vi "BrightfieldControl.vi"() -> ()   [LabVIEW 2019]
doc: "high-level user control for uc480/ThorCam DCx camera. include MouseMove, this allows mouse click to move stage motor capabilities"
uses:
  <vilib>/Utility/miscctls.llb/LVPoint32TypeDef.ctl
  C:/Program Files/Thorlabs/Scientific Imaging/DCx Camera Support/Develop/DotNet/uc480DotNet.dll
  System.Drawing
  System.Windows.Forms
panel:
  out "Coords":T1
  out "# in queue":i32
  in  "motor move?":bool
  out "mouse click":string
  out "mm value w":dbl
  out "mm value h":dbl
  in  "micron/pixel":dbl=2.0
  in  "stop video loop":bool
  out "current video state":string="wait for init"
  in  "save video?":bool
  in  "mode":i32(ring)=128 items=["BGRA8Packed"=0, "BGR8Packed"=1, "BGR565Packed"=2, "BGR5Packed"=3, "Mono8"=6, "SensorRaw8"=11, "UYVYPacked"=12, "UYVYMonoPacked"=13, "UYVYBayerPacked"=14, "CBYCRYPacked"=23, "BGRY8Packed"=24, "BGR10Packed"=25, "Mono12"=26, "SensorRaw12"=27, "Mono16"=28, "SensorRaw16"=29, "BGR12Unpacked"=30, "BGRA12Unpacked"=31, "Jpeg"=32, "SensorRaw10"=33, "Mono10"=34, "BGR10Unpacked"=35, "RGBA8Packed"=128, "RGB8Packed"=129, "RGBY8Packed"=152, "RGB10Packed"=153, "RGB12Unpacked"=158, "RGBA12Unpacked"=159, "RGB10Unpacked"=163, "RGB8Planar"=8321, "PreferPackedSourceFormat"=16384]
  out "img saved to:":string
  in  "Folder path save":path
  in  "PictureBox":refnum<k24>(container)
  in  "Stop Button":bool
  in  "Image filename save":string="D:\\Victor Sun\\optical trap control\\output_test\\test"
  in  "save snapshot?":bool
  in  "Pixelclock":i32(slide)=24 scale=5.0..43.0
  in  "Framerate":dbl(slide)=7.0 scale=5.0..14.0
  in  "Exposure time":dbl(slide)=30.0 scale=1.0..70.0
  out "SerialNumber":string
  in  "s32Cam":i32
  # "MouseMove"
  # "trying to figure out to use .net video \nto get .avi"
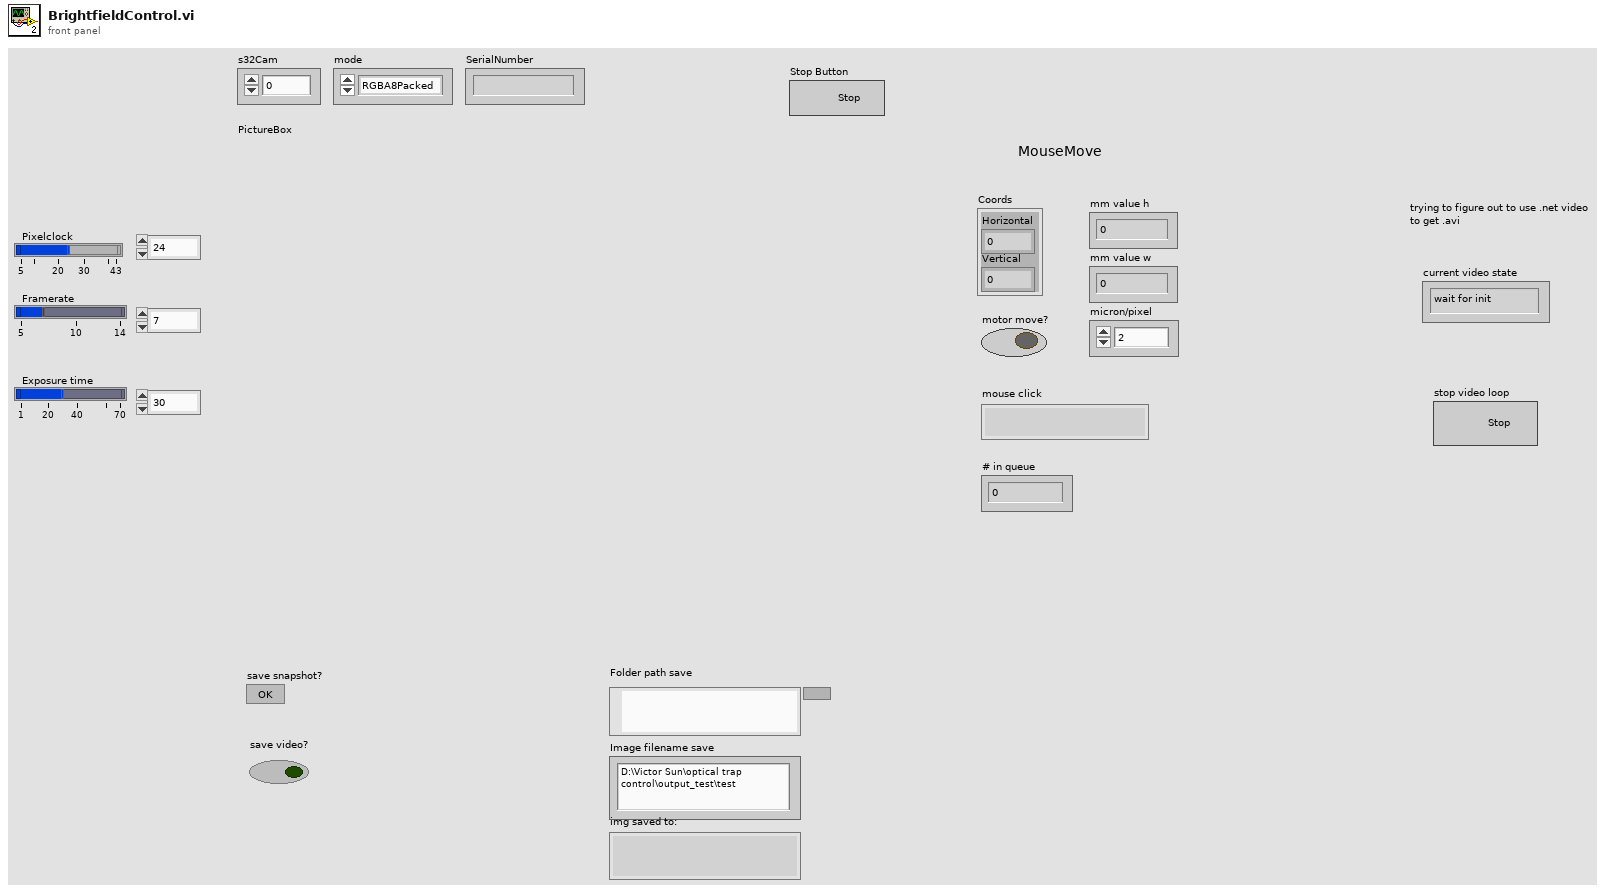
[diagram p1: front panel]
types:
  T1 = typedef "LVPoint32TypeDef.ctl" = cluster{"Horizontal":i32, "Vertical":i32}
  T2 = enum16{"wait for init", "init video", "wait for write", "write frame", "close video"}
  T3 = typedef "IMAQ AVI2 Refnum.ctl" = refnum<k20>
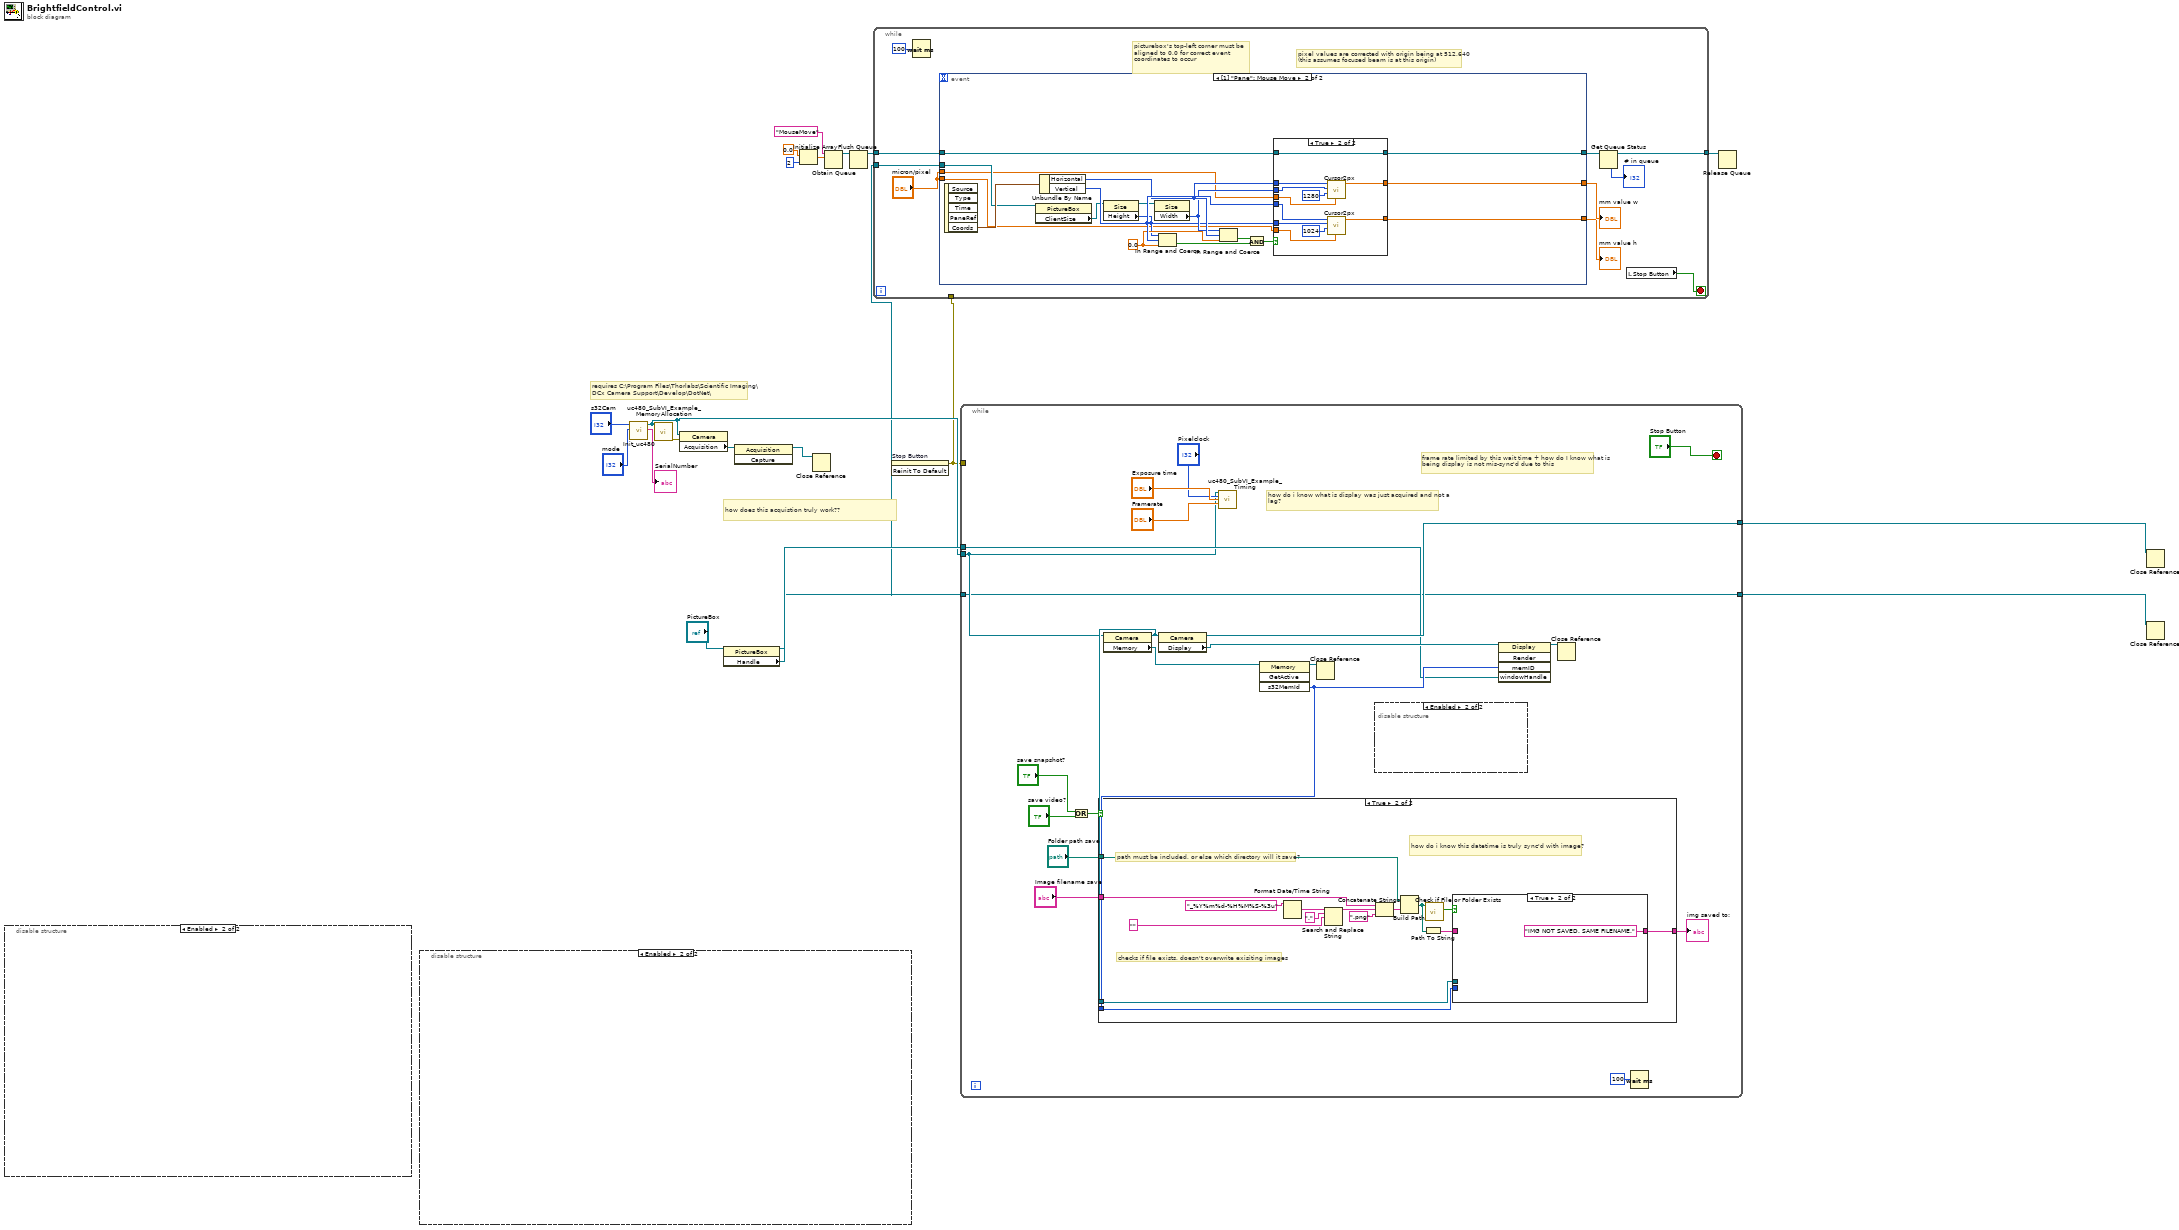
[diagram p0: block diagram]
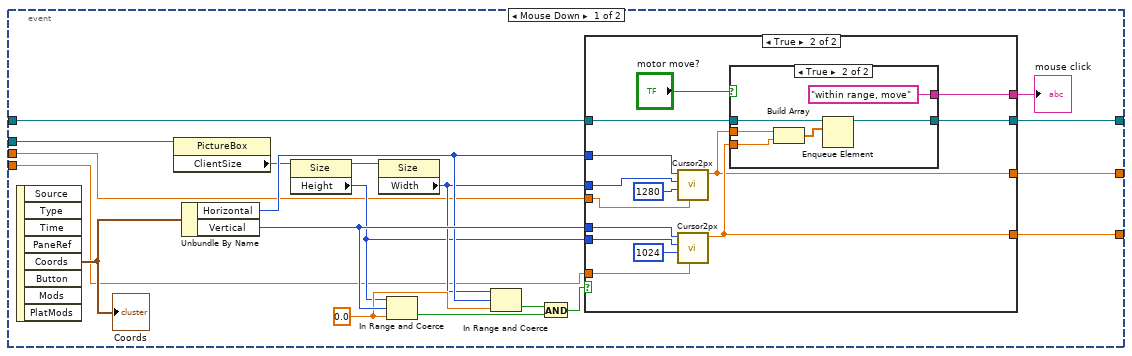
[diagram p2: hidden frame]
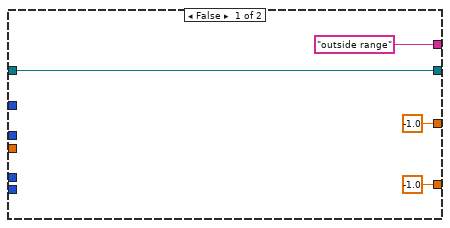
[diagram p3: hidden frame]
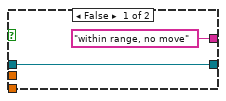
[diagram p4: hidden frame]
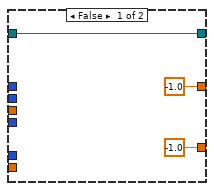
[diagram p5: hidden frame]
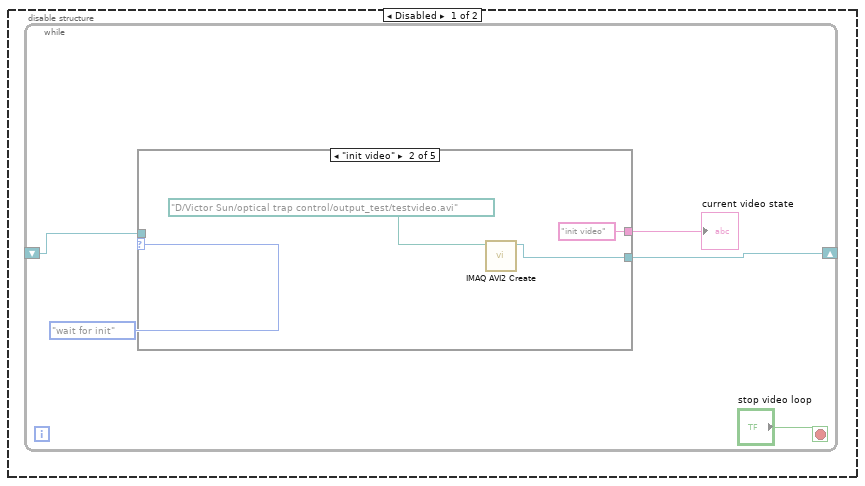
[diagram p6: hidden frame]
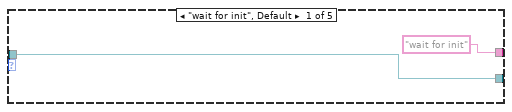
[diagram p7: hidden frame]
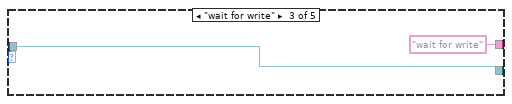
[diagram p8: hidden frame]
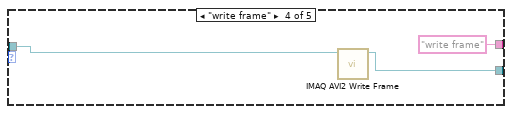
[diagram p9: hidden frame]
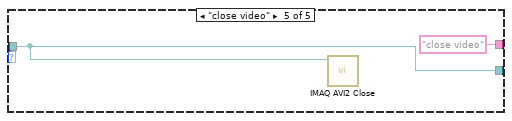
[diagram p10: hidden frame]
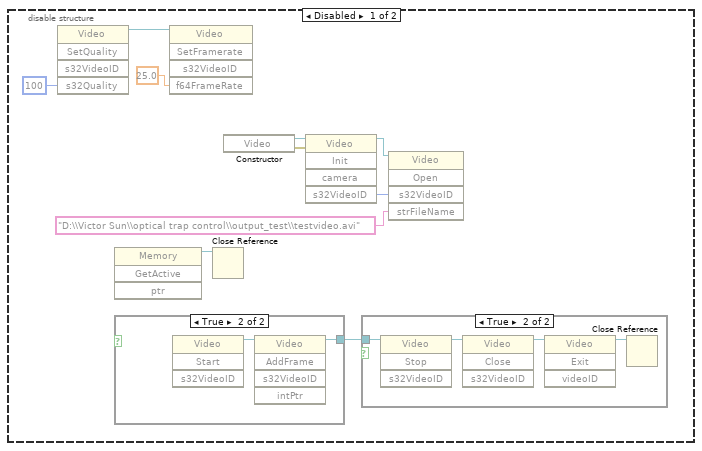
[diagram p11: hidden frame]
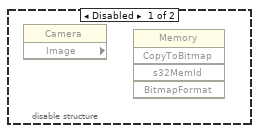
[diagram p14: hidden frame]
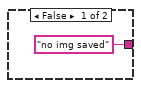
[diagram p15: hidden frame]
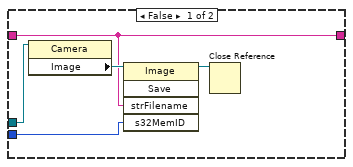
[diagram p16: hidden frame]
diagram:
  # "requires C:\\Program Files\\Thorlabs\\Scientific Imaging\\DCx Camera Support\\Develop\\DotNet\\"
  # "how does this acquistion truly work??"
  n1 = disable-structure shown="Enabled" {
    frame Disabled {
      n2 = invoke class="Video" method="SetQuality"("s32Quality"=100) -> (reference out=w25:refnum<k24>)  [unwired: 4 in, 4 out]
      n3 = invoke class="Memory" method="GetActive"() -> (reference out=w22:refnum<k24>)  [unwired: 4 in, 3 out]
      n4 = case shown="True" {
        selector: _ -> [_ _]
        tunnel: [_ w35] -> w21
        frame False {
        }
        frame True {
          n5 = invoke class="Video" method="Start"() -> (reference out=w36:refnum<k24>)  [unwired: 4 in, 3 out]
          n6 = invoke class="Video" method="AddFrame"(reference=w36) -> (reference out=w35:refnum<k24>)  [unwired: 4 in, 4 out]
        }
      }
      n7 = invoke class="Video" method="SetFramerate"(reference=w25, "f64FrameRate"=25.0) -> ()  [unwired: 3 in, 5 out]
      n8 = Close Reference(reference=w22) -> ()  [unwired: 1 in, 1 out]
      n9 = constructor class="Video"() -> (reference out=w28:refnum<k24>, error out=w29:errorcluster)  [unwired: 3 in, 1 out]
      n10 = invoke class="Video" method="Init"(reference=w28, error in=w29) -> (reference out=w26:refnum<k24>, "s32VideoID"=w30:i32)  [unwired: 3 in, 3 out]
      n11 = case shown="True" {
        selector: _ -> [_ _]
        tunnel: w21 -> [_ w34]
        frame False {
        }
        frame True {
          n12 = invoke class="Video" method="Stop"(reference=w34) -> (reference out=w33:refnum<k24>)  [unwired: 3 in, 3 out]
          n13 = invoke class="Video" method="Close"(reference=w33) -> (reference out=w32:refnum<k24>)  [unwired: 3 in, 3 out]
          n14 = invoke class="Video" method="Exit"(reference=w32) -> (reference out=w31:refnum<k24>)  [unwired: 3 in, 3 out]
          n15 = Close Reference(reference=w31) -> ()  [unwired: 1 in, 1 out]
        }
      }
      n16 = invoke class="Video" method="Open"(reference=w26, "s32VideoID"=w30, "strFileName"="D:\\Victor Sun\\optical trap control\\output_test\\testvideo.avi") -> ()  [unwired: 2 in, 5 out]
    }
    frame Enabled {
    }
  }
  n17 = disable-structure shown="Enabled" {
    frame Disabled {
      n18 = while {
        shift-right: [w38] -> _
        shift-left: _ -> [w37]
        stop <- "stop video loop" stop-if-true
        n19 = case shown="\"init video\"" T2."wait for init" {
          tunnel: ["wait for init" "init video" "wait for write" "write frame" "close video"] -> w40
          tunnel: [w42 w44 w47 w49 w52] -> w38
          tunnel: w37 -> [w42 _ w47 w50 w52]
          frame "wait for init", Default {
          }
          frame "init video" {
            n20 = call "IMAQ AVI2 Create"("AVI Path"=path "D:/Victor Sun/optical trap control/output_test/testvideo.avi") -> ("AVI Refnum"=w44:T3)  [unwired: 9 in, 1 out]
          }
          frame "wait for write" {
          }
          frame "write frame" {
            n21 = call "IMAQ AVI2 Write Frame"("AVI Refnum"=w50) -> ("AVI Refnum (duplicate)"=w49:T3)  [unwired: 8 in, 2 out]
          }
          frame "close video" {
            n22 = call "IMAQ AVI2 Close"("AVI Refnum"=w52) -> ()  [unwired: 10 in, 1 out]
          }
        }
        "current video state" <- w40
      }
    }
    frame Enabled {
    }
  }
  n23 = call "Init_uc480.vi"("mode"="mode", "s32Cam"="s32Cam") -> ("SerialNumber"=→"SerialNumber":string, ".NET Refnum out"=w11:refnum<k24>)  [unwired: 8 in]
  n24 = call <instrlib>:"uc480_SubVI_Example_MemoryAllocation.vi"(".NET (Reference)"=w11) -> ("Error Out"=w12:errorcluster)  [unwired: 14 in, 4 out]
  n25 = property class="Camera"(reference=w11, error in=w12) -> ("Acquisition"=w13:refnum<k24>)  [unwired: 2 out]
  n26 = property class="PictureBox"(reference="PictureBox") -> (reference out=w9:refnum<k24>, "Handle"=w15:refnum<k24>)  [unwired: 1 in, 1 out]
  n27 = invoke class="Acquisition" method="Capture"(reference=w13) -> (reference out=w14:refnum<k24>)  [unwired: 2 in, 2 out]
  n28 = Initialize Array(0.0 ("element"), 2 ("dimension size")) -> (w5:dbl[])
  n29 = Close Reference(reference=w14) -> ()  [unwired: 1 in, 1 out]
  n30 = Obtain Queue(name (unnamed)="MouseMove", element data type=w5) -> (queue out=w3:refnum<queue>)  [unwired: 3 in, 2 out]
  n31 = Flush Queue(queue=w3) -> (queue out=w4:refnum<queue>)  [unwired: 1 in, 2 out]
  n32 = invoke on="Stop Button" class="Bool (strict)" method="Reinit To Default"() -> (error out=w1:errorcluster)  [unwired: 3 in, 2 out]
  n33 = while {
    tunnel: w9 -> [w62]
    tunnel: w4 -> [w61]
    tunnel: [w58] -> w2
    tunnel: w1 -> [_]
    stop <- w54 stop-if-true
    # "picturebox's top-left corner must be aligned to 0,0 for correct event coordinates to occur"
    # "pixel values are corrected with origin being at 512,640\n(this assumes focused beam is at this origin)"
    n34 = Wait (ms)(milliseconds to wait=u32 100) -> ()  [unwired: 1 out]
    n35 = event shown="[1] \"Pane\": Mouse Move" {
      selector: _ -> [_ _]
      dyn-events: _ -> [_ _]
      timeout: _ -> [_ _]
      tunnel: w62 -> [w72 w117]
      tunnel: w61 -> [w69 w114]
      tunnel: [w68 w113] -> w59
      tunnel: [w67 w112] -> w57
      tunnel: [w66 w111] -> w56
      tunnel: "micron/pixel" -> [w65 w110]
      tunnel: "micron/pixel" -> [w64 w109]
      event Mouse Down {
        w76 = 0.0 ("lower limit")
        n36 = event-data() -> ("Coords"=w82:T1)  [unwired: 1 in, 7 out]
        "Coords" <- w82
        n37 = property class="PictureBox"(reference=w72) -> ("ClientSize"=w73:refnum<k24>)  [unwired: 1 in, 2 out]
        n38 = Unbundle By Name(w82) -> ("Horizontal"=w77:i32, "Vertical"=w80:i32)
        n39 = property class="Size"(reference=w73) -> (reference out=w74:refnum<k24>, "Height"=w70:i32)  [unwired: 1 in, 1 out]
        n40 = property class="Size"(reference=w74) -> ("Width"=w71:i32)  [unwired: 1 in, 2 out]
        n41 = In Range and Coerce(upper limit=w70, x=w80, lower limit=w76) -> (In Range?=w79:bool)  [unwired: 1 out]
        n42 = In Range and Coerce(upper limit=w71, x=w77, lower limit=w76) -> (In Range?=w78:bool)  [unwired: 1 out]
        n43 = And(x=w78, y=w79) -> (x .and. y?=w81:bool)
        n44 = case shown="True" w81 {
          tunnel: w80 -> [_ w100]
          tunnel: w70 -> [_ w99]
          tunnel: w71 -> [_ w96]
          tunnel: w77 -> [_ w95]
          tunnel: ["outside range" ("mouse click") w93] -> w75
          tunnel: w69 -> [w85 w92]
          tunnel: [w85 w91] -> w68
          tunnel: [-1.0 ("mm value") w90] -> w66
          tunnel: [-1.0 ("mm value") w89] -> w67
          tunnel: w65 -> [_ w88]
          tunnel: w64 -> [_ w87]
          frame False {
          }
          frame True {
            n45 = call "Cursor2px.vi"("micron/pixel"=w87, "Image dimension"=1280, "Picturebox dimension"=w96, "Cursor dimension"=w95) -> ("mm value"=w89:dbl)  [unwired: 6 in, 1 out]
            n46 = call "Cursor2px.vi"("micron/pixel"=w88, "Image dimension"=1024, "Picturebox dimension"=w99, "Cursor dimension"=w100) -> ("mm value"=w90:dbl)  [unwired: 6 in, 1 out]
            n47 = case shown="True" "motor move?" {
              tunnel: ["within range, no move" ("mouse click") "within range, move" ("mouse click")] -> w93
              tunnel: w89 -> [_ w107]
              tunnel: w90 -> [_ w106]
              tunnel: w92 -> [w101 w104]
              tunnel: [w101 w103] -> w91
              frame False {
              }
              frame True {
                n48 = Build Array(w107, w106) -> (w105:dbl[])
                n49 = Enqueue Element(queue=w104, element=w105) -> (queue out=w103:refnum<queue>)  [unwired: 2 in, 2 out]
              }
            }
          }
        }
        "mouse click" <- w75
      }
      event Mouse Move {
        w120 = 0.0 ("lower limit")
        n50 = event-data() -> ("Coords"=w126:T1)  [unwired: 1 in, 4 out]
        n51 = property class="PictureBox"(reference=w117) -> ("ClientSize"=w118:refnum<k24>)  [unwired: 1 in, 2 out]
        n52 = Unbundle By Name(w126) -> ("Horizontal"=w121:i32, "Vertical"=w124:i32)
        n53 = property class="Size"(reference=w118) -> (reference out=w119:refnum<k24>, "Height"=w115:i32)  [unwired: 1 in, 1 out]
        n54 = property class="Size"(reference=w119) -> ("Width"=w116:i32)  [unwired: 1 in, 2 out]
        n55 = In Range and Coerce(upper limit=w115, x=w124, lower limit=w120) -> (In Range?=w123:bool)  [unwired: 1 out]
        n56 = In Range and Coerce(upper limit=w116, x=w121, lower limit=w120) -> (In Range?=w122:bool)  [unwired: 1 out]
        n57 = And(x=w122, y=w123) -> (x .and. y?=w125:bool)
        n58 = case shown="True" w125 {
          tunnel: w124 -> [_ w140]
          tunnel: w115 -> [_ w139]
          tunnel: w116 -> [_ w136]
          tunnel: w121 -> [_ w135]
          tunnel: w114 -> [w129 w132]
          tunnel: [w129 w132] -> w113
          tunnel: [-1.0 ("mm value") w134] -> w111
          tunnel: [-1.0 ("mm value") w133] -> w112
          tunnel: w110 -> [_ w131]
          tunnel: w109 -> [_ w130]
          frame False {
          }
          frame True {
            n59 = call "Cursor2px.vi"("micron/pixel"=w130, "Image dimension"=1280, "Picturebox dimension"=w136, "Cursor dimension"=w135) -> ("mm value"=w133:dbl)  [unwired: 6 in, 1 out]
            n60 = call "Cursor2px.vi"("micron/pixel"=w131, "Image dimension"=1024, "Picturebox dimension"=w139, "Cursor dimension"=w140) -> ("mm value"=w134:dbl)  [unwired: 6 in, 1 out]
          }
        }
      }
    }
    "mm value h" <- w56
    "mm value w" <- w57
    n61 = Get Queue Status(queue=w59) -> (queue out=w58:refnum<queue>, # elements in queue=→"# in queue":i32)  [unwired: 2 in, 6 out]
    n62 = local read "Stop Button"() -> (w54:bool)
  }
  n63 = while {
    tunnel: w9 -> [w141]
    tunnel: [w141] -> w18
    tunnel: w11 -> [w145]
    tunnel: w15 -> [w153]
    tunnel: [w156] -> w17
    tunnel: w1 -> [_]
    stop <- "Stop Button" stop-if-true
    # "frame rate limited by this wait time + how do I know what is being display is not mis-sync'd due to this"
    # "how do i know what is display was just acquired and not a lag?"
    n64 = Or(x="save snapshot?", y="save video?") -> (x .or. y?=w146:bool)
    n65 = property class="Camera"(reference=w145) -> (reference out=w155:refnum<k24>, "Memory"=w159:refnum<k24>)  [unwired: 1 in, 1 out]
    n66 = property class="Camera"(reference=w155) -> (reference out=w156:refnum<k24>, "Display"=w158:refnum<k24>)  [unwired: 1 in, 1 out]
    n67 = call <instrlib>:"uc480_SubVI_Example_Timing.vi"(".NET (Reference)"=w145, "Pixelclock"="Pixelclock", "Exposure time"="Exposure time", "Framerate"="Framerate") -> ()  [unwired: 8 in, 4 out]
    n68 = invoke class="Memory" method="GetActive"(reference=w159) -> (reference out=w144:refnum<k24>, "s32MemId"=w154:i32)  [unwired: 3 in, 2 out]
    n69 = case shown="True" w146 {
      tunnel: w155 -> [_ w177]
      tunnel: w154 -> [_ w176]
      tunnel: ["no img saved" ("snapshot filename") w172] -> w149
      tunnel: "Folder path save" -> [_ w164]
      tunnel: "Image filename save" -> [_ w163]
      frame False {
      }
      frame True {
        # "path must be included, or else which directory will it save?"
        # "checks if file exists, doesn't overwrite exisiting images"
        # "how do i know this datetime is truly sync'd with image?"
        n70 = Format Date/Time String(time format string (%c)="_%Y%m%d-%H%M%S-%3u") -> (date/time string=w171:string)  [unwired: 2 in]
        n71 = Search and Replace String(input string=w171, search string=".", replace string="" ("replace string (\"\")")) -> (result string=w167:string)  [unwired: 5 in, 3 out]
        n72 = Concatenate Strings(w163, w167, ".png" ("result string")) -> (w166:string)
        n73 = Build Path(base path=w164, name or relative path=w166) -> (appended path=w174:path)
        n74 = Path To String(path=w174) -> (string=w175:string)
        n75 = call <vilib>:"Check if File or Folder Exists.vi"("path"=w174) -> ("file or folder exists?"=w173:bool)  [unwired: 8 in, 2 out]
        n76 = case shown="True" w173 {
          tunnel: w177 -> [w180 _]
          tunnel: w176 -> [w179 _]
          tunnel: w175 -> [w178 _]
          tunnel: [w178 "IMG NOT SAVED. SAME FILENAME."] -> w172
          frame False {
            n77 = property class="Camera"(reference=w180) -> ("Image"=w182:refnum<k24>)  [unwired: 1 in, 2 out]
            n78 = invoke class="Image" method="Save"(reference=w182, "strFilename"=w178, "s32MemID"=w179) -> (reference out=w181:refnum<k24>)  [unwired: 2 in, 4 out]
            n79 = Close Reference(reference=w181) -> ()  [unwired: 1 in, 1 out]
          }
          frame True {
          }
        }
      }
    }
    "img saved to:" <- w149
    n80 = Close Reference(reference=w144) -> ()  [unwired: 1 in, 1 out]
    n81 = disable-structure shown="Enabled" {
      frame Disabled {
        n82 = property class="Camera" props=["Image"]() -> ()  [unwired: 2 in, 3 out]
        n83 = invoke class="Memory" method="CopyToBitmap"() -> ()  [unwired: 5 in, 5 out]
      }
      frame Enabled {
      }
    }
    n84 = invoke class="Display" method="Render"(reference=w158, "memID"=w154, "windowHandle"=w153) -> (reference out=w157:refnum<k24>)  [unwired: 2 in, 4 out]
    n85 = Close Reference(reference=w157) -> ()  [unwired: 1 in, 1 out]
    n86 = Wait (ms)(milliseconds to wait=u32 100) -> ()  [unwired: 1 out]
  }
  n87 = Release Queue(queue=w2) -> ()  [unwired: 2 in, 3 out]
  n88 = Close Reference(reference=w17) -> ()  [unwired: 1 in, 1 out]
  n89 = Close Reference(reference=w18) -> ()  [unwired: 1 in, 1 out]
